vi "TCPIP Connect.vi"(8 "error in (no error)":errorcluster, 9 "Port":i32, 10 "TCP address":string) -> (0 "error out":errorcluster, 3 "CreateIp":refnum<k24>)   [LabVIEW 2022 SP3]
uses:
  C:/Users/carl2/Downloads/Modbus Demo v1.3/Modbus Demo v1.3/DLL/Modbus.dll
  DLL/Modbus.dll
  C:/Users/carl2/Downloads/Modbus Demo v1.3/Modbus Demo v1.3/DLL/LabVIEW_CSLib.dll
  DLL/LabVIEW_CSLib.dll
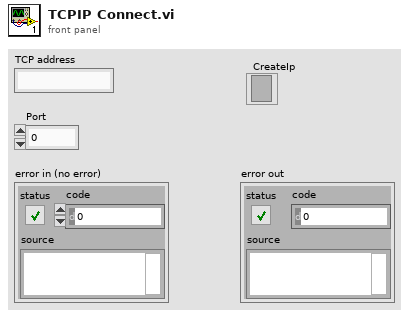
[diagram p1: front panel]
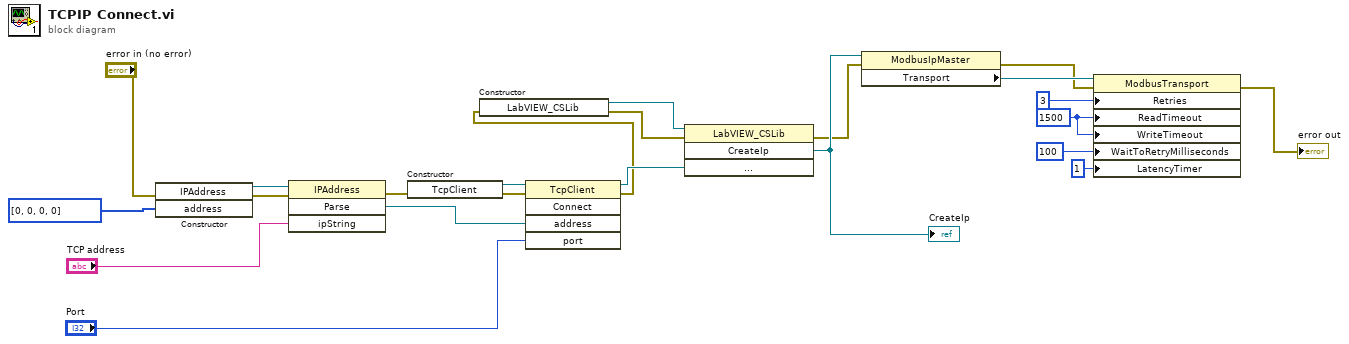
[diagram p0: block diagram]
diagram:
  w10 = 1500 ("ReadTimeout")
  n1 = constructor class="IPAddress"(error in="error in (no error)", "address"=u8[] [0, 0, 0, 0]) -> (reference out=w16:refnum<k24>, error out=w22:errorcluster)  [unwired: 2 in, 2 out]
  n2 = invoke class="IPAddress" method="Parse"(reference=w16, error in=w22, "ipString"="TCP address") -> (error out=w21:errorcluster, "Parse"=w19:refnum<k24>)  [unwired: 1 in, 2 out]
  n3 = constructor class="TcpClient"(error in=w21) -> (reference out=w15:refnum<k24>, error out=w17:errorcluster)  [unwired: 2 in, 1 out]
  n4 = invoke class="TcpClient" method="Connect"(reference=w15, error in=w17, "address"=w19, "port"="Port") -> (reference out=w5:refnum<k24>, error out=w2:errorcluster)  [unwired: 1 in, 3 out]
  n5 = constructor class="LabVIEW_CSLib"(error in=w2) -> (reference out=w13:refnum<k24>, error out=w1:errorcluster)  [unwired: 2 in, 1 out]
  n6 = invoke class="LabVIEW_CSLib" method="CreateIp"(reference=w13, error in=w1, "tcpClient"=w5) -> (error out=w6:errorcluster, "CreateIp"=w12:refnum<k24>)  [unwired: 1 in, 2 out]
  "CreateIp" <- w12
  n7 = property class="ModbusIpMaster"(reference=w12, error in=w6) -> (error out=w7:errorcluster, "Transport"=w8:refnum<k24>)  [unwired: 1 out]
  n8 = property class="ModbusTransport"(reference=w8, error in=w7, "Retries"=3, "ReadTimeout"=w10, "WriteTimeout"=w10, "WaitToRetryMilliseconds"=100, "LatencyTimer"=1) -> (error out=→"error out":errorcluster)  [unwired: 1 out]
